vi "ApplyPostScale.vi"(8 "error in (no error)":errorcluster, 10 "Waveform Array":sgl[][](array[numeric]), 11 "DAQ Actor in":refnum<class "DAQ Actor.lvclass">) -> (0 "error out":errorcluster, 2 "Waveform Array":sgl[][](array[numeric]), 3 "DAQ Actor Out":refnum<class "DAQ Actor.lvclass">)   [LabVIEW 2018, in "Data Acquisition.lvlib" / "DAQ Actor.lvclass"]
doc: "Post process temperature and rtd measurement types by providing a scale and offset.\nSteve Karcher 3/12/2012"
uses:
  DAQ Actor.lvclass
  DAQ Actor.lvclass/DAQ Actor.ctl
  Class DAQ Task/DAQ Task.lvclass/DAQ Task.ctl
  Class DAQ Task/Read All Channels.vi
  Measurements/Class Channel/Channel.lvclass
  Class DAQ Task/DAQ Task.lvclass
panel:
  # "slk change 3/12/2012\nvi added to post process temperature and rtd measurement types for scaling and offset"
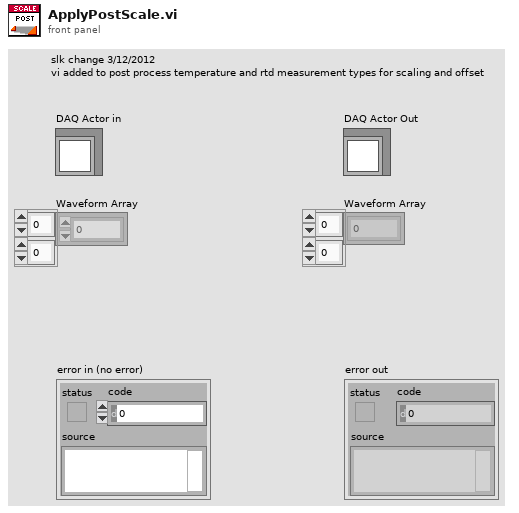
[diagram p1: front panel]
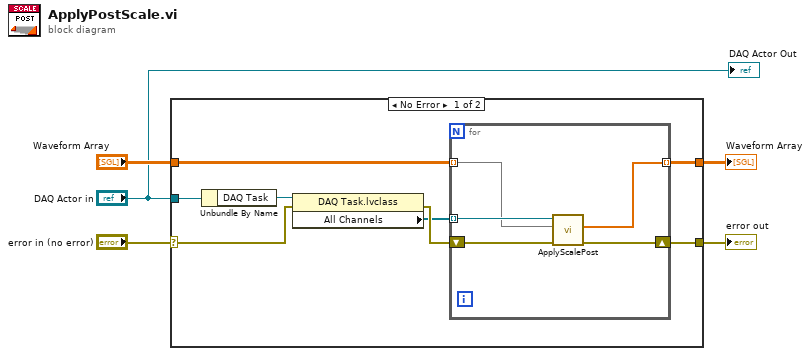
[diagram p0: block diagram]
diagram:
  n1 = case shown="No Error" "error in (no error)" {
    selector: "error in (no error)" -> [w7 w20]
    tunnel: "Waveform Array" -> [w13 w19]
    tunnel: [w12 w19] -> w4
    tunnel: [w11 w20] -> w3
    tunnel: "DAQ Actor in" -> [w10 _]
    frame No Error {
      n2 = Unbundle By Name(w10) -> ("DAQ Task"=w9:refnum<class "DAQ Task.lvclass">)
      n3 = property class="DAQ Task.lvclass"(reference=w9, error in=w7) -> (error out=w8:errorcluster, "All Channels"=w6:refnum<class "Channel.lvclass">[])  [unwired: 1 out]
      n4 = for {
        tunnel: w6 -> [w17] mode=indexing
        shift-right: [w15] -> w11
        shift-left: w8 -> [w18]
        tunnel: w13 -> [w16] mode=indexing
        tunnel: [w14] -> w12 mode=indexing
        n5 = call-dynamic "ApplyScalePost.vi"("error in (no error)"=w18, "Y Array"=w16, "Channel in"=w17) -> ("error out"=w15:errorcluster, "Y Array"=w14:sgl[])  [unwired: 6 in, 1 out]
      }
    }
    frame Error {
    }
  }
  "Waveform Array" <- w4
  "error out" <- w3
  "DAQ Actor Out" <- "DAQ Actor in"
